vi "uTTA_SetCH_Description.vi"(8 "error in":errorcluster, 9 "Channel No":i32, 10 "Channel Description":T1, 11 "VISA Refnum in":refnum<visa-resource-name>) -> (0 "error out":errorcluster, 2 "Received":string, 3 "VISA Refnum out":refnum<visa-resource-name>)   [LabVIEW 2021]
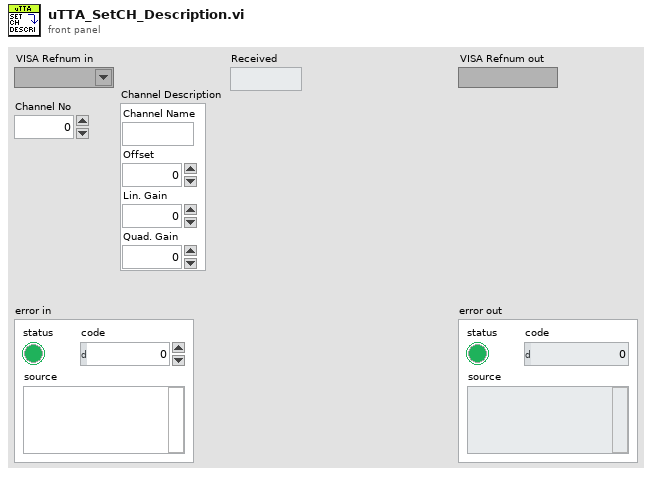
[diagram p1: front panel]
types:
  T1 = cluster{"Channel Name":string, "Offset":dbl, "Lin. Gain":dbl, "Quad. Gain":dbl}
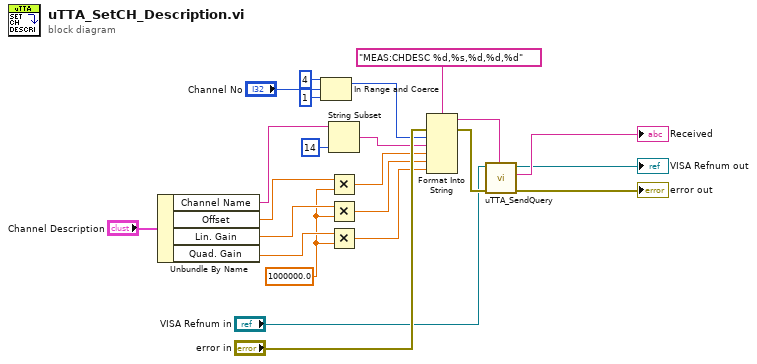
[diagram p0: block diagram]
diagram:
  w1 = 1000000.0 ("y")
  n1 = Unbundle By Name("Channel Description") -> ("Channel Name"=w8:string, "Offset"=w7:dbl, "Lin. Gain"=w3:dbl, "Quad. Gain"=w2:dbl)
  n2 = In Range and Coerce(upper limit=4, x="Channel No", lower limit=1) -> (coerced(x)=w12:i32)  [unwired: 1 out]
  n3 = String Subset(string=w8, length (rest)=14 ("length (rest)")) -> (substring=w14:string)  [unwired: 1 in]
  n4 = Multiply(x=w7, y=w1) -> (x*y=w6:dbl)
  n5 = Multiply(x=w3, y=w1) -> (x*y=w5:dbl)
  n6 = Multiply(x=w2, y=w1) -> (x*y=w4:dbl)
  n7 = Format Into String(format string="MEAS:CHDESC %d,%s,%d,%d,%d", error in="error in", w12, w14, w6, w5, w4) -> (resulting string=w20:string, error out=w22:errorcluster)  [unwired: 1 in]
  n8 = call "uTTA_SendQuery.vi"("Send String"=w20, "error in (no error)"=w22, "VISA Refnum in"="VISA Refnum in") -> ("error out"=→"error out":errorcluster, "Received"=→"Received":string, "VISA Refnum out"=→"VISA Refnum out":refnum<visa-resource-name>)  [unwired: 6 in]
